vi "tsdiag_can_test_present.vi"(8 "error in (no error)":errorcluster, 9 "response required?":bool=TRUE, 10 "ADiagModuleIndex":i32, 11 "路径输入":path) -> (0 "error out":errorcluster, 1 "Succes？":bool, 2 "Return Type":i32, 3 "路径输出":path)   [LabVIEW 2014]
doc: "3E服务，诊断仪在线。"
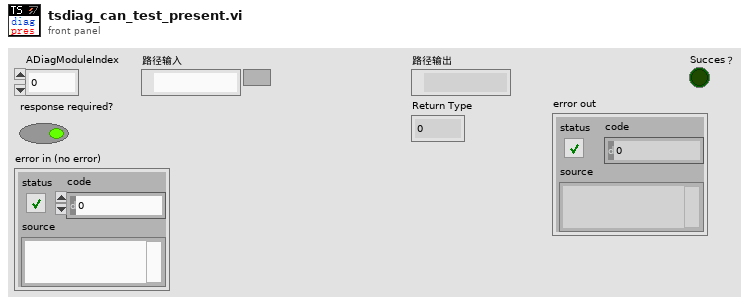
[diagram p1: front panel]
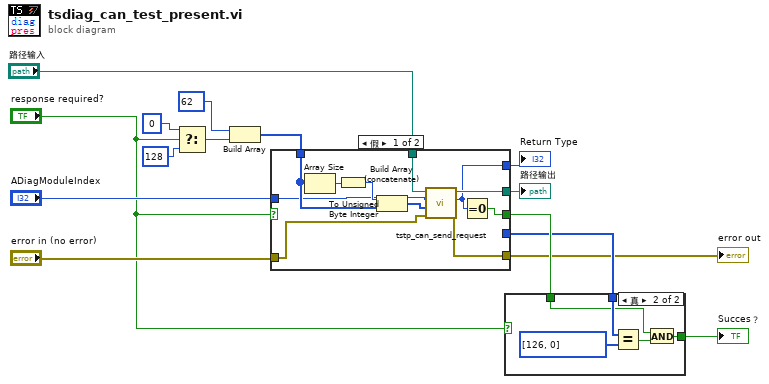
[diagram p0: block diagram]
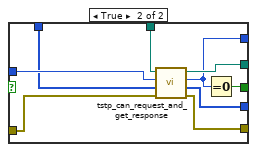
[diagram p3: hidden frame]
diagram:
  n1 = Select(t=u8 0, s="response required?", f=u8 128) -> (s? t:f=w11:u8)
  n2 = Build Array(u8 62, w11) -> (w10:u8[])
  n3 = case shown="假" "response required?" {
    tunnel: "ADiagModuleIndex" -> [w22 w33]
    tunnel: w10 -> [w25 w32]
    tunnel: "error in (no error)" -> [w20 w35]
    tunnel: [w19 w34] -> w5
    tunnel: [_ w29] -> w6
    tunnel: [w18 w30] -> w7
    tunnel: "路径输入" -> [w23 w31]
    tunnel: [w17 w28] -> w2
    tunnel: [w16 w27] -> w1
    frame False {
      n4 = Array Size(array=w25) -> (size(s)=w26:i32)
      n5 = To Unsigned Byte Integer(number=w26) -> (unsigned 8bit integer=w24:u8)
      n6 = Build Array (concatenate)(w24, w25) -> (w21:u8[])
      n7 = call "tstp_can_send_request.vi"("error in (no error)"=w20, "Data"=w21, "ADiagModuleIndex"=w22, "路径输入"=w23) -> ("error out"=w19:errorcluster, "return"=w16:i32, "路径输出"=w17:path)  [unwired: 5 in]
      n8 = Equal To 0?(x=w16) -> (x = 0?=w18:bool)
    }
    frame True {
      n9 = call "tstp_can_request_and_get_response.vi"("错误输入（无错误）"=w35, "AReqDataArray"=w32, "ADiagModuleIndex"=w33, "path"=w31) -> ("错误输出"=w34:errorcluster, "Diagnostic response"=w29:u8[], "Return Type"=w27:i32, "path out"=w28:path)  [unwired: 4 in]
      n10 = Equal To 0?(x=w27) -> (x = 0?=w30:bool)
    }
  }
  "error out" <- w5
  "路径输出" <- w2
  "Return Type" <- w1
  n11 = case shown="真" "response required?" {
    tunnel: w6 -> [_ w41]
    tunnel: w7 -> [w36 w38]
    tunnel: [w36 w37] -> w4
    frame False {
    }
    frame True {
      n12 = Equal?(x=w41, y=u8[] [126, 0]) -> (x = y?=w39:bool)
      n13 = And(x=w38, y=w39) -> (x .and. y?=w37:bool)
    }
  }
  "Succes？" <- w4
